vi "Catch Nested Value Update.vi"(8 "error in (no error)":errorcluster, 10 "Nested Value Update Msg":refnum<class "Nested Value Update Msg.lvclass">, 11 "TopLevelApplication In":refnum<class "ConcreteViewModel.lvclass">) -> (0 "error out":errorcluster, 3 "TopLevelApplication Out":refnum<class "ConcreteViewModel.lvclass">)   [LabVIEW 2020, in "TopLevelApplication.lvlib" / "ConcreteViewModel.lvclass"]
doc: "<License>\nCopyright © 2017 Composed Systems, LLC | All rights reserved\nwww.composed.io\n\nAuthor: Ethan Stern <ethan.stern@composed.io>\n\nThis software is provided \"AS IS\" WITHOUT WARRANTIES, either express or implied, AND IS FOR EDUCATIONAL PURPOSES ONLY.\n</License>"
uses:
  ConcreteViewModel.lvclass
  C:/Git/mva-framework/modules/mva-viewable/Source/IViewModel/IViewModel/IViewModel.lvclass
  C:/Git/mva-framework/modules/mva-viewable/Source/IViewable/IViewable/IViewable.lvclass
  modules/mva-viewable/Source/IViewable/IViewable Messages/Catch Nested Value Change Msg/Nested Value Update Msg.lvclass
  modules/mva-viewable/Source/IViewable/IViewable Messages/Catch Nested Value Change Msg/Nested Value Update Msg.lvclass/Nested Value Update Msg.ctl
  modules/mva-core/Source/IObserver/IObserver/IObserver.lvclass/IObserver.ctl
  modules/mva-viewable/Source/IViewModel/IViewModel/IViewModel.lvclass/IViewModel.ctl
  modules/mva-core/Source/IMediator/PublishRequest/PublishRequest.lvclass/PublishRequest.ctl
  modules/mva-core/Source/IMediator/IMediator Messages/Publish Msg/Publish Msg.lvclass/Publish Msg.ctl
  modules/composed-af-messages/Source/RoundTripMessage/RoundTripMessage.lvclass/RoundTripMessage.ctl
  <vilib>/ActorFramework/Message Enqueuer/Message Enqueuer.lvclass/Message Enqueuer.ctl
  modules/mva-core/Source/IMediator/IMediator Messages/Publish Msg/Send Pre-Addressed Publish.vi
  modules/mva-core/Source/IObserver/IObserver/Read Unique ID.vi
  modules/mva-core/Source/IMediator/PublishRequest/Pack Publish Request.vi
  modules/composed-af-messages/Source/RoundTripMessage/Return Round-Trip Message.vi
  <vilib>/ActorFramework/Message Enqueuer/Enqueue.vi
  modules/mva-viewable/Source/IViewModel/IViewModel/IViewModel.lvclass
  C:/Git/mva-framework/modules/mva-core/Source/IObserver/IObserver/IObserver.lvclass
  modules/mva-core/Source/IMediator/IMediator Messages/Publish Msg/Publish Msg.lvclass
  C:/Git/mva-framework/modules/composed-af-messages/Source/RoundTripMessage/RoundTripMessage.lvclass
  modules/composed-af-messages/Source/RoundTripMessage/RoundTripMessage.lvclass
  C:/Program Files (x86)/National Instruments/LabVIEW 2020/vi.lib/ActorFramework/Message/Message.lvclass
  <vilib>/Utility/error.llb/Error Cluster From Error Code.vi
  <vilib>/ActorFramework/Message Priority Queue/Priority Enqueue.vi
  modules/mva-core/Source/IMediator/PublishRequest/PublishRequest.lvclass
  <vilib>/Utility/Data Type/NI_Data Type.lvlib
  Source/DialogBox/OneButtonDialogBox/OneButtonDialogBox.lvclass
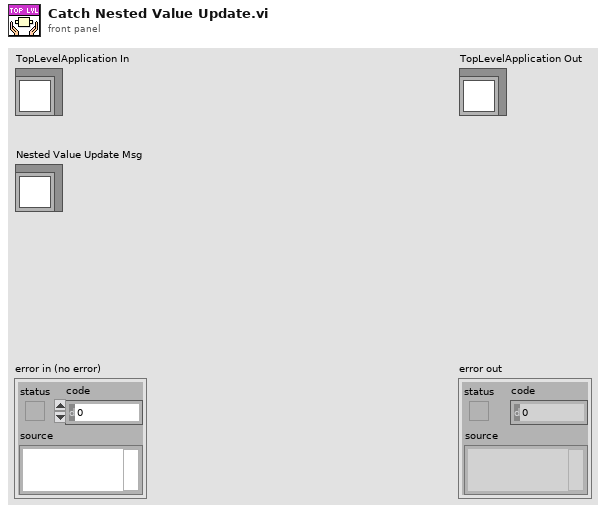
[diagram p1: front panel]
types:
  T1 = typedef "NI_Data Type.lvlib/Data Type.ctl" = enum8{"Invalid Type", "Void", "I8", "I16", "I32", "I64", "U8", "U16", "U32", "U64", "Single Float", "Double Float", "Extended Float", "Single Complex", "Double Complex", "Extended Complex", "Enum U8", "Enum U16", "Enum U32", "Enum U64", "Single Float With Unit", "Double Float With Unit", "Extended Float With Unit", "Single Complex with Unit", "Double Complex with Unit", "Extended Complex with Unit", "Boolean", "String", "Path", "Picture", "Tag", "Array", "Cluster", "Variant", "LV Variant", "Waveform", "Timestamp", "Digital Waveform", "Digital Data", "ExpressData", "Refnum", "External Data", "VI", "Poly VI", "LabVIEW Class Instance", "Fixed Point", "Set Collection", "Map Collection"}
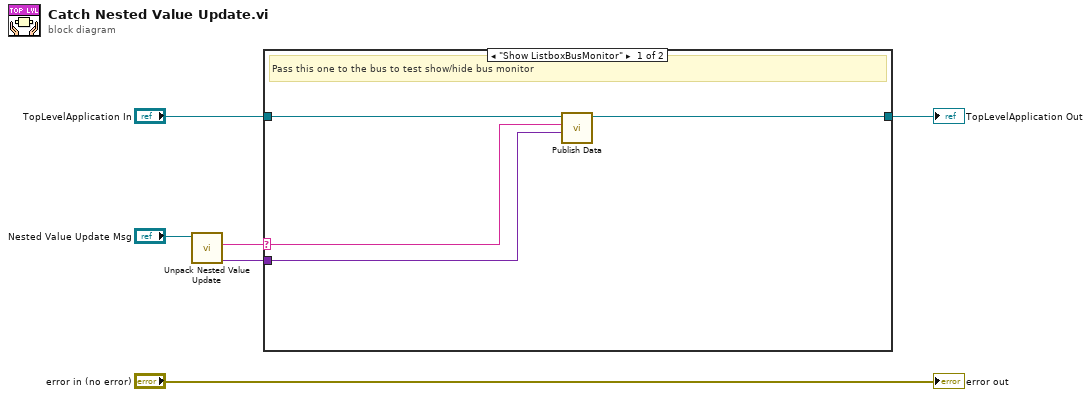
[diagram p0: block diagram]
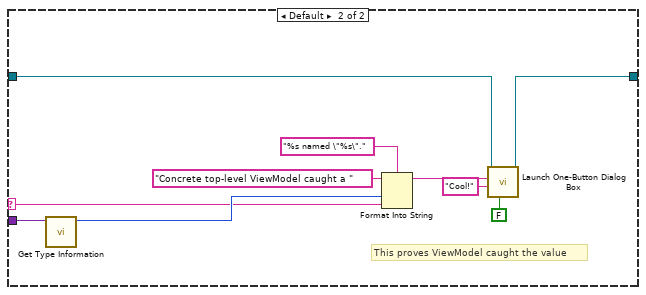
[diagram p2: hidden frame]
diagram:
  n1 = call "Unpack Nested Value Update.vi"("Nested Value Update Msg"="Nested Value Update Msg") -> ("Value"=w4:variant, "Datum Name"=w3:string)  [unwired: 8 in, 1 out]
  n2 = case shown="\"Show ListboxBusMonitor\"" w3 {
    selector: w3 -> [w8 w13]
    tunnel: w4 -> [w7 w14]
    tunnel: "TopLevelApplication In" -> [w10 w12]
    tunnel: [w9 w11] -> w1
    frame "Show ListboxBusMonitor" {
      # "Pass this one to the bus to test show/hide bus monitor"
      n3 = call "Publish Data.vi"("Data to Publish"=w7, "Datum Name"=w8, "IViewModel In"=w10) -> ("IViewModel Out"=w9:refnum<class "ConcreteViewModel.lvclass">)  [unwired: 7 in, 1 out]
    }
    frame Default {
      # "This proves ViewModel caught the value"
      n4 = call <vilib>:"Get Type Information.vi"("variant"=w14) -> ("type"=w16:T1)  [unwired: 6 in, 4 out]
      n5 = Format Into String(format string="%s named \"%s\".", initial string="Concrete top-level ViewModel caught a ", w16, w13) -> (resulting string=w18:string)  [unwired: 1 in, 1 out]
      n6 = call "Launch One-Button Dialog Box.vi"("Modal? (T)"=FALSE, "Button Text (OK)"="Cool!", "Message Text"=w18, "Dialog Launcher"=w12) -> ("Dialog Launcher Out"=w11:refnum<class "ConcreteViewModel.lvclass">)  [unwired: 6 in, 1 out]
    }
  }
  "TopLevelApplication Out" <- w1
  "error out" <- "error in (no error)"
